vi "Set Channel String Offset.vi"(8 "error in (no error)":errorcluster, 10 "string offset":u64, 11 "channel in":T1={"core"={"name"="", "units"="V", "engine data type"=enum."DBL", "string data type"=enum."DBL", "string offset"=0}, "component settings"=[]} {"core"."string offset" format="%d bytes"}) -> (0 "error out":errorcluster, 3 "channel out":T1={"core"={"name"="", "units"="V", "engine data type"=enum."DBL", "string data type"=enum."DBL", "string offset"=0}, "component settings"=[]} {"core"."string offset" format="%d bytes"})   [LabVIEW 2017, in "DSF Core.lvlib" / "Configuration Session.lvclass"]
uses:
  Configuration Session.lvclass
  Typedefs/DSF Engine Channel Configuration.ctl
  Typedefs/DSF Core Channel Configuration.ctl
  Typedefs/DSF Data Type.ctl
  Typedefs/DSF Settings Info.ctl
  Typedefs/DSF Version Info.ctl
  DSF Core.lvlib
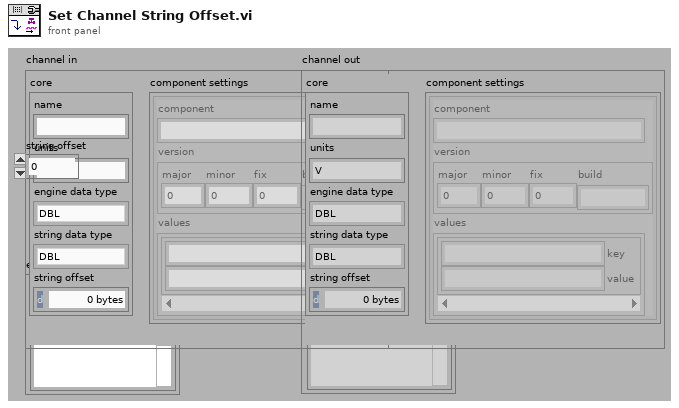
[diagram p1: front panel]
types:
  T1 = typedef "DSF Core.lvlib/DSF Engine Channel Configuration.ctl" = cluster{"core":T2, "component settings":T4[]}
  T2 = typedef "DSF Core.lvlib/DSF Core Channel Configuration.ctl" = cluster{"name":string, "units":string, "engine data type":T3, "string data type":T3, "string offset":u64}
  T3 = typedef "DSF Core.lvlib/DSF Data Type.ctl" = enum8{"Bool", "SGL", "DBL", "I8", "I16", "I32", "I64", "U8", "U16", "U32", "U64"}
  T4 = typedef "DSF Core.lvlib/DSF Settings Info.ctl" = cluster{"component":string, "version":T5, "values":cluster{"key":string, "value":string}[]}
  T5 = typedef "DSF Core.lvlib/DSF Version Info.ctl" = cluster{"major":u32, "minor":u32, "fix":u32, "build":string}
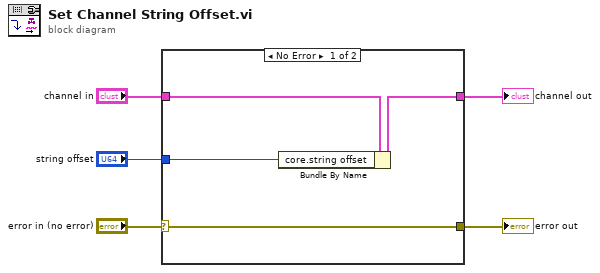
[diagram p0: block diagram]
diagram:
  n1 = case shown="No Error" "error in (no error)" {
    selector: "error in (no error)" -> [w7 w11]
    tunnel: [w7 w11] -> w5
    tunnel: [w8 w10] -> w2
    tunnel: "channel in" -> [w9 w10]
    tunnel: "string offset" -> [w6 _]
    frame No Error {
      n2 = Bundle By Name(cluster=w9, "core.string offset"=w6) -> (w8:T1)
    }
    frame Error {
    }
  }
  "error out" <- w5
  "channel out" <- w2
